vi "Position Set Invert Values All.vi"(8 "Error":errorcluster, 9 "FwdBk(F) LR(T)":bool, 11 "RobotDriveDevRef":T1) -> (0 "Error Out":errorcluster, 3 "RobotDriveDevRef Out":T1)   [LabVIEW 2017, in "MechamunDrive.lvlib"]
uses:
  MechamunDrive.lvlib
  <vilib>/Rock Robotics/WPI/RobotDrive/WPI_RobotDriveDevRef.ctl
  <vilib>/Rock Robotics/WPI/MotorControl/WPI_MotorControlDeviceRef.ctl
  <vilib>/Rock Robotics/WPI/MotorControl/WPI_MotorControlType.ctl
  <vilib>/Rock Robotics/SystemInterfaces/DIO/FPGA_DIOPWMChannel.ctl
  <vilib>/Rock Robotics/WPI/PWM/WPI_PWMDeadband.ctl
  <vilib>/Rock Robotics/SystemInterfaces/DIO/FPGA_DIOChannel.ctl
  <vilib>/Rock Robotics/WPI/RobotDrive/WPI_RobotDriveMotorSelectorEnum.ctl
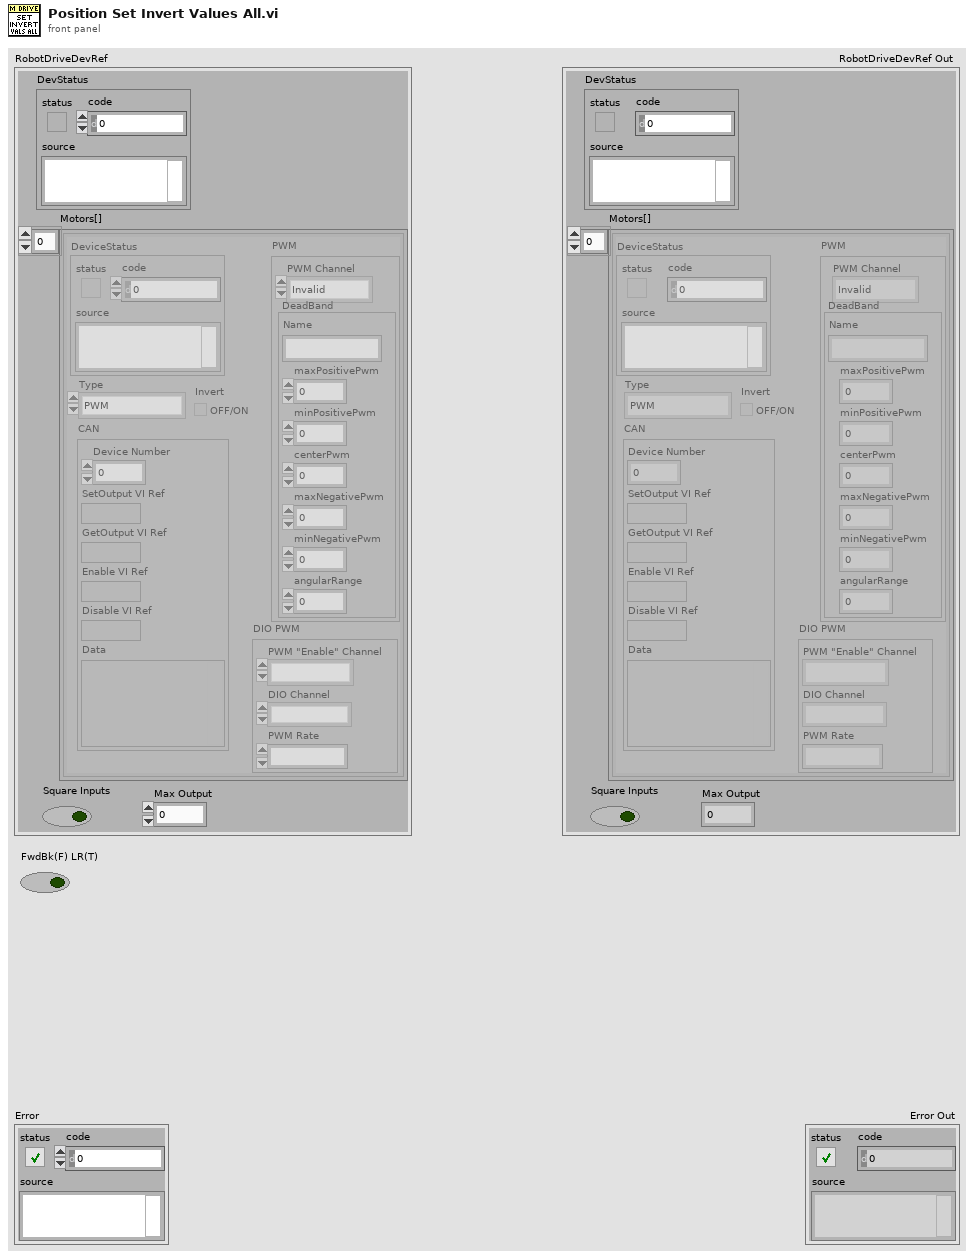
[diagram p1: front panel]
types:
  T1 = typedef "WPI_RobotDriveDevRef.ctl" = cluster{"DevStatus":errorcluster, "Motors[]":T2[], "Square Inputs":bool, "Max Output":dbl}
  T2 = typedef "WPI_MotorControlDeviceRef.ctl" = cluster{"DeviceStatus":errorcluster, "Type":T3, "PWM":cluster{"PWM Channel":T4, "DeadBand":T5}, "CAN":cluster{"Device Number":u8, "SetOutput VI Ref":variant, "GetOutput VI Ref":variant, "Enable VI Ref":variant, "Disable VI Ref":variant, "Data":variant}, "Invert":bool, "DIO PWM":cluster{"PWM \"Enable\" Channel":T4, "DIOChannel":T6, "PWM Rate":dbl}}
  T3 = typedef "WPI_MotorControlType.ctl" = enum16{"PWM", "CAN", "DIO PWM"}
  T4 = typedef "FPGA_DIOPWMChannel.ctl" = enum8{"PWM 0", "PWM 1", "PWM 2", "PWM 3", "PWM 4", "PWM 5", "PWM 6", "PWM 7", "PWM 8", "PWM 9", "PWM MXP 0", "PWM MXP 1", "PWM MXP 2", "PWM MXP 3", "PWM MXP 4", "PWM MXP 5", "PWM MXP 6", "PWM MXP 7", "PWM MXP 8", "PWM MXP 9", "Invalid"}
  T5 = typedef "WPI_PWMDeadband.ctl" = cluster{"Name":string, "maxPositivePwm":i32, "minPositivePwm":i32, "centerPwm":i32, "maxNegativePwm":i32, "minNegativePwm":i32, "angularRange":u16}
  T6 = typedef "FPGA_DIOChannel.ctl" = enum8{"DIO 0", "DIO 1", "DIO 2", "DIO 3", "DIO 4", "DIO 5", "DIO 6", "DIO 7", "DIO 8", "DIO 9", "DIO MXP 0", "DIO MXP 1", "DIO MXP 2", "DIO MXP 3", "DIO MXP 4", "DIO MXP 5", "DIO MXP 6", "DIO MXP 7", "DIO MXP 8", "DIO MXP 9", "DIO MXP 10", "DIO MXP 11", "DIO MXP 12", "DIO MXP 13", "DIO MXP 14", "DIO MXP 15", "SPI Port CS1", "SPI Port CS2", "SPI Port CS3", "SPI Port MISO", "SPI Port MOSI", "Invalid"}
  T7 = typedef "WPI_RobotDriveMotorSelectorEnum.ctl" = enum16{"Rear Left Motor", "Rear Right Motor", "Front Left Motor", "Front Right Motor"}
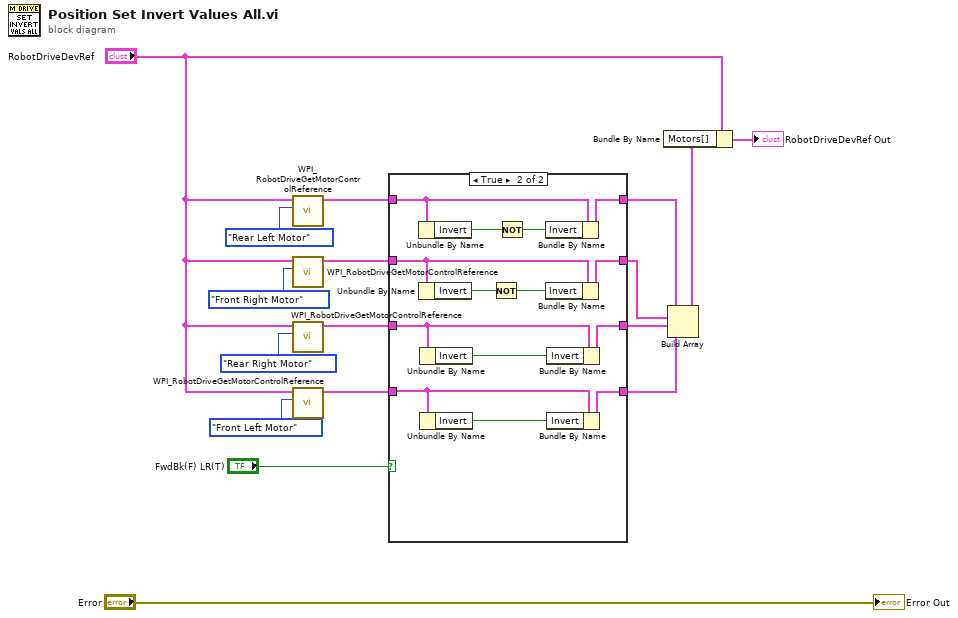
[diagram p0: block diagram]
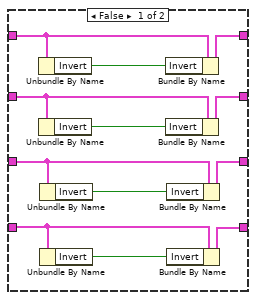
[diagram p2: hidden frame]
diagram:
  n1 = call <vilib>:"WPI_RobotDriveGetMotorControlReference.vi"("MotorIndex"=WPI_RobotDriveMotorSelectorEnum."Rear Left Motor", "RobotDriveDevRef"="RobotDriveDevRef") -> ("MotorControlDeviceRef"=w11:T2)  [unwired: 9 out]
  n2 = call <vilib>:"WPI_RobotDriveGetMotorControlReference.vi"("MotorIndex"=WPI_RobotDriveMotorSelectorEnum."Front Right Motor", "RobotDriveDevRef"="RobotDriveDevRef") -> ("MotorControlDeviceRef"=w10:T2)  [unwired: 9 out]
  n3 = call <vilib>:"WPI_RobotDriveGetMotorControlReference.vi"("MotorIndex"=WPI_RobotDriveMotorSelectorEnum."Rear Right Motor", "RobotDriveDevRef"="RobotDriveDevRef") -> ("MotorControlDeviceRef"=w9:T2)  [unwired: 9 out]
  n4 = call <vilib>:"WPI_RobotDriveGetMotorControlReference.vi"("MotorIndex"=WPI_RobotDriveMotorSelectorEnum."Front Left Motor", "RobotDriveDevRef"="RobotDriveDevRef") -> ("MotorControlDeviceRef"=w8:T2)  [unwired: 9 out]
  n5 = case shown="True" "FwdBk(F) LR(T)" {
    tunnel: w11 -> [w28 w42]
    tunnel: w10 -> [w25 w39]
    tunnel: w9 -> [w22 w36]
    tunnel: w8 -> [w19 w33]
    tunnel: [w29 w43] -> w3
    tunnel: [w24 w38] -> w4
    tunnel: [w21 w35] -> w5
    tunnel: [w18 w32] -> w6
    frame False {
      n6 = Unbundle By Name(w28) -> ("Invert"=w27:bool)
      n7 = Unbundle By Name(w25) -> ("Invert"=w26:bool)
      n8 = Unbundle By Name(w22) -> ("Invert"=w23:bool)
      n9 = Unbundle By Name(w19) -> ("Invert"=w20:bool)
      n10 = Bundle By Name(cluster=w28, "Invert"=w27) -> (w29:T2)
      n11 = Bundle By Name(cluster=w25, "Invert"=w26) -> (w24:T2)
      n12 = Bundle By Name(cluster=w22, "Invert"=w23) -> (w21:T2)
      n13 = Bundle By Name(cluster=w19, "Invert"=w20) -> (w18:T2)
    }
    frame True {
      n14 = Unbundle By Name(w42) -> ("Invert"=w41:bool)
      n15 = Unbundle By Name(w39) -> ("Invert"=w40:bool)
      n16 = Unbundle By Name(w36) -> ("Invert"=w37:bool)
      n17 = Unbundle By Name(w33) -> ("Invert"=w34:bool)
      n18 = Not(x=w40) -> (.not. x?=w31:bool)
      n19 = Not(x=w41) -> (.not. x?=w30:bool)
      n20 = Bundle By Name(cluster=w42, "Invert"=w30) -> (w43:T2)
      n21 = Bundle By Name(cluster=w39, "Invert"=w31) -> (w38:T2)
      n22 = Bundle By Name(cluster=w36, "Invert"=w37) -> (w35:T2)
      n23 = Bundle By Name(cluster=w33, "Invert"=w34) -> (w32:T2)
    }
  }
  n24 = Build Array(w3, w4, w5, w6) -> (w2:T2[])
  n25 = Bundle By Name(cluster="RobotDriveDevRef", "Motors[]"=w2) -> (→"RobotDriveDevRef Out":T1)
  "Error Out" <- "Error"
